vi "Run Step.vi"(8 "error in (no error)":errorcluster, 9 "result allocation":T1, 10 "parameters":T1, 11 "Wait Step in":refnum<class "Wait Step.lvclass">) -> (0 "error out":errorcluster, 1 "results":T1, 2 "parameter allocation":T1, 3 "Wait Step out":refnum<class "Wait Step.lvclass">)   [LabVIEW 2015, in "Wait Step.lvclass"]
uses:
  Wait Step.lvclass
  <vilib>/NI/Tag Bus/table/data table.ctl
  classes/Step/Execution/StepState.ctl
  classes/Step/Execution/Step Status.ctl
  classes/Step/Execution/Step Flow Control.ctl
  Wait Step.lvclass/Wait Step.ctl
  classes/Step/Execution/Step.lvclass
  <vilib>/NI/Tag Bus/table/data table.lvlib
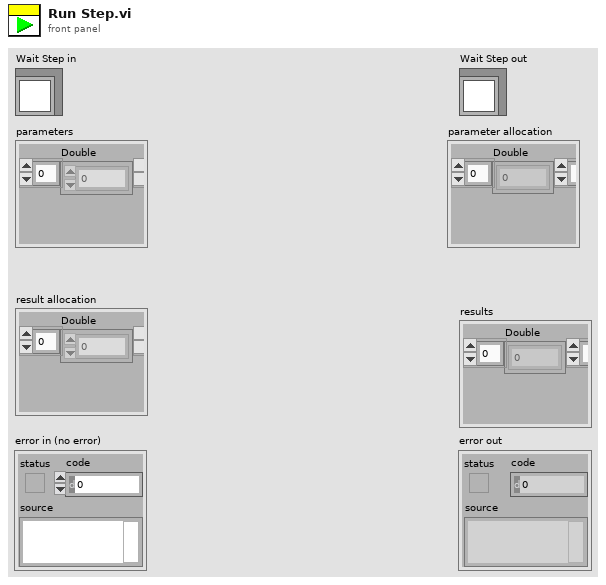
[diagram p1: front panel]
types:
  T1 = typedef "tag bus.lvlib/data table.lvlib/data table.ctl" = cluster{"Double":dbl[], "Single":sgl[], "I64":i64[], "I32":i32[], "I16":i16[], "I8":i8[], "U64":u64[], "U32":u32[], "U16":u16[], "U8":u8[], "Boolean":bool[], "String":string[], "Array of Double":cluster{"DBL Array":dbl[]}[], "Array of Single":cluster{"SGL Array":sgl[]}[], "Array of I64":cluster{"I64 Array":i64[]}[], "Array of I32":cluster{"I32 Array":i32[]}[], "Array of I16":cluster{"I16 Array":i16[]}[], "Array of I8":cluster{"I8 Array":i8[]}[], "Array of U64":cluster{"U64 Array":u64[]}[], "Array of U32":cluster{"U32 Array":u32[]}[], "Array of U16":cluster{"U16 Array":u16[]}[], "Array of U8":cluster{"U8 Array":u8[]}[], "Array of Boolean":cluster{"Boolean Array":bool[]}[], "Array of String":cluster{"String Array":string[]}[]}
  T2 = typedef "Step.lvclass/Step Status.ctl" = enum16{"Start", "Passed", "Failed", "Error", "Done", "Terminated", "Skipped", "Running"}
  T3 = typedef "Step.lvclass/StepState.ctl" = cluster{"Step State":T2, "Flow Control":T4, "Jump Index":i32, "Done":bool}
  T4 = typedef "Step.lvclass/Step Flow Control.ctl" = enum16{"Next Step", "Jump"}
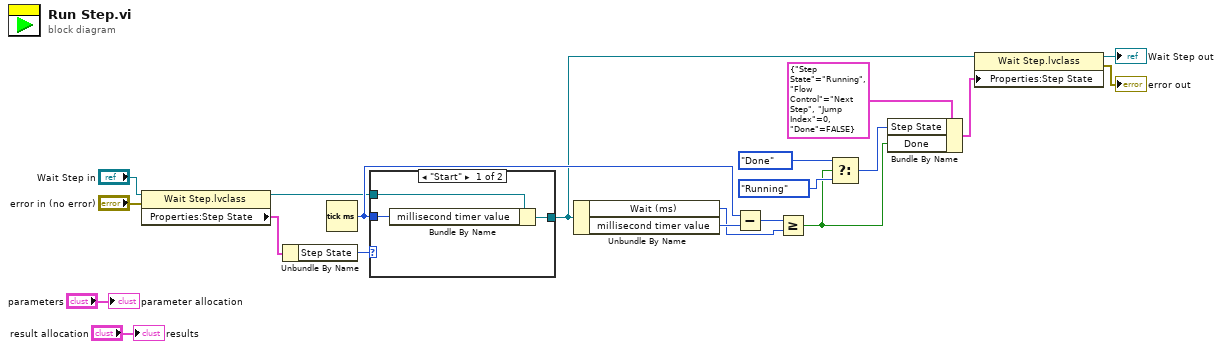
[diagram p0: block diagram]
diagram:
  n1 = property class="Wait Step.lvclass"(reference="Wait Step in", error in="error in (no error)") -> (reference out=w10:refnum<class "Wait Step.lvclass">, "Properties:Step State"=w8:T3)  [unwired: 1 out]
  n2 = Unbundle By Name(w8) -> ("Step State"=w7:T2)
  n3 = Tick Count (ms)() -> (millisecond timer value=w20:u32)
  n4 = case shown="\"Start\"" w7 {
    tunnel: w20 -> [w21 _]
    tunnel: w10 -> [w23 w24]
    tunnel: [w22 w24] -> w11
    frame "Start" {
      n5 = Bundle By Name(cluster=w23, "millisecond timer value"=w21) -> (w22:refnum<class "Wait Step.lvclass">)
    }
    frame "Skipped", Default {
    }
  }
  n6 = Unbundle By Name(w11) -> ("Wait (ms)"=w17:u32, "millisecond timer value"=w19:u32)
  n7 = Subtract(x=w20, y=w19) -> (x-y=w18:u32)
  n8 = Greater Or Equal?(x=w18, y=w17) -> (x >= y?=w2:bool)
  n9 = Select(t=Step_Status."Done" ("Step State"), s=w2, f=Step_Status."Running" ("Step State")) -> (s? t:f=w3:T2)
  n10 = Bundle By Name(cluster=T3 {"Step State"=enum."Running", "Flow Control"=enum."Next Step", "Jump Index"=0, "Done"=FALSE} ("f"), "Step State"=w3, "Done"=w2) -> (w1:T3)
  n11 = property class="Wait Step.lvclass"(reference=w11, "Properties:Step State"=w1) -> (reference out=→"Wait Step out":refnum<class "Wait Step.lvclass">, error out=→"error out":errorcluster)  [unwired: 1 in]
  "parameter allocation" <- "parameters"
  "results" <- "result allocation"
